vi "Auth Check & Log.vi"(8 "error in":errorcluster, 10 "User Cred":T1, 11 "Authenticated Data":string[][](array[string])) -> (0 "error out":errorcluster, 1 "User":string, 2 "Role Out":string, 3 "Verify Auth":bool)   [LabVIEW 2022 SP3]
uses:
  <vilib>/Utility/file.llb/Write Delimited Spreadsheet (string).vi
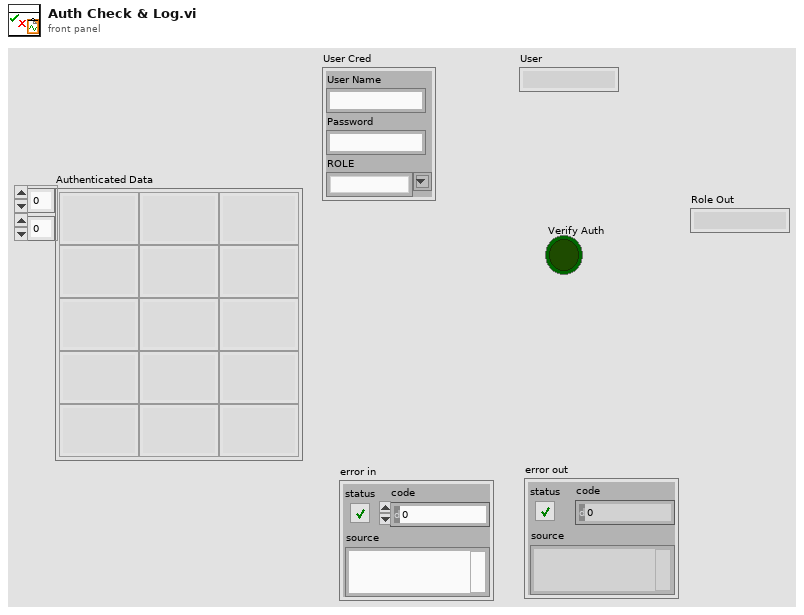
[diagram p1: front panel]
types:
  T1 = cluster{"User Name":string, "Password":string, "ROLE":string}
  T2 = typedef "SeCrTs-file folder ctl.ctl" = cluster{"Datalog path":path, "Configuration path":path, "Signal list path":path, "Sub vi's":path, "Authentication":path, "Sequence":path, "Event Log":path, "CS Error log":path, "RT Error Log":path}
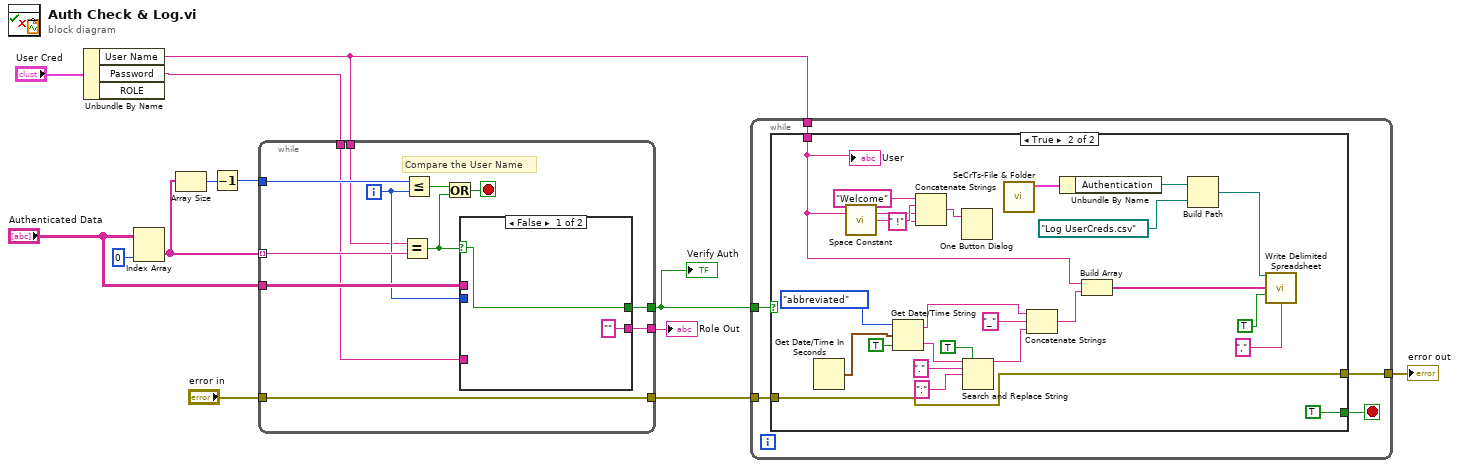
[diagram p0: block diagram]
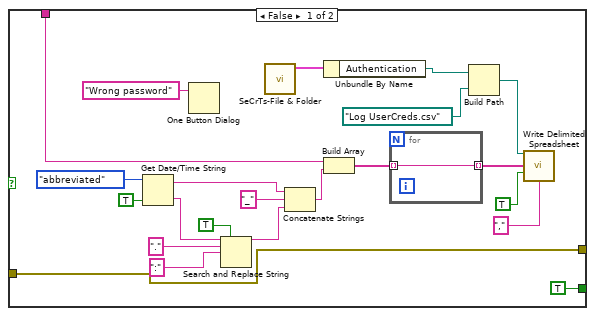
[diagram p2: hidden frame]
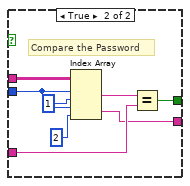
[diagram p3: hidden frame]
diagram:
  n1 = Unbundle By Name("User Cred") -> ("User Name"=w8:string, "Password"=w7:string)  [unwired: 1 out]
  n2 = Index Array(array="Authenticated Data", index (col)=0 ("disabled index (col)")) -> (element=w10:string[])  [unwired: 1 in]
  n3 = Array Size(array=w10) -> (size(s)=w12:i32)
  n4 = Decrement(x=w12) -> (x-1=w11:i32)
  n5 = while {
    tunnel: w11 -> [w25]
    tunnel: w10 -> [w24] mode=indexing
    tunnel: "Authenticated Data" -> [w20]
    tunnel: [w18] -> w9
    tunnel: w8 -> [w16]
    tunnel: w7 -> [w17]
    tunnel: "error in" -> [w15]
    tunnel: [w15] -> w5
    tunnel: [w14] -> w1
    i -> [w19]
    stop <- w21 stop-if-true
    # "Compare the User Name"
    n6 = Equal?(x=w16, y=w24) -> (x = y?=w22:bool)
    n7 = Less Or Equal?(x=w25, y=w19) -> (x <= y?=w23:bool)
    n8 = Or(x=w23, y=w22) -> (x .or. y?=w21:bool)
    n9 = case shown="False" w22 {
      selector: w22 -> [w27 _]
      tunnel: w20 -> [_ w35]
      tunnel: w19 -> [_ w29]
      tunnel: [w27 w32] -> w18
      tunnel: w17 -> [_ w31]
      tunnel: ["" ("String") w28] -> w14
      frame False {
      }
      frame True {
        # "Compare the Password"
        n10 = Index Array(array=w35, index (row) #1=w29, index (col) #1=1 ("disabled index (col)"), index (row) #2=w29, index (col) #2=2 ("index (col)")) -> (element #1=w33:string, element #2=w28:string)
        n11 = Equal?(x=w33, y=w31) -> (x = y?=w32:bool)
      }
    }
  }
  "Verify Auth" <- w9
  "Role Out" <- w1
  n12 = while {
    tunnel: w9 -> [w40]
    tunnel: w8 -> [w38]
    tunnel: w5 -> [w37]
    tunnel: [w36] -> w4
    stop <- w39 stop-if-true
    n13 = case shown="True" w40 {
      tunnel: [TRUE TRUE] -> w39
      tunnel: w38 -> [w44 w65]
      tunnel: w37 -> [w45 w72]
      tunnel: [w45 w72] -> w36
      frame False {
        # "Log user credentials including username,Password and  login time"
        n14 = Get Date/Time String(date format (0)=enum16{"short", "long", "abbreviated"}."abbreviated", want seconds? (F)=TRUE) -> (date string=w60:string, time string=w58:string)  [unwired: 1 in]
        n15 = One Button Dialog(message="Wrong password") -> ()  [unwired: 1 in, 1 out]
        n16 = Search and Replace String(replace all?=TRUE ("replace all? (F)"), input string=w58, search string=".", replace string=":" ("replace string (\"\")")) -> (result string=w59:string)  [unwired: 4 in, 3 out]
        n17 = call "SeCrTs-File & Folder.vi"() -> ("File Output"=w41:T2)  [unwired: 10 in, 1 out]
        n18 = Concatenate Strings(w60, "_" ("string"), w59) -> (w43:string)
        n19 = Unbundle By Name(w41) -> ("Authentication"=w42:path)
        n20 = Build Array(w44, w43) -> (w61:string[])
        n21 = for {
          tunnel: w61 -> [w63] mode=indexing
          tunnel: [w63] -> w62 mode=indexing
        }
        n22 = Build Path(base path=w42, name or relative path=path "Log UserCreds.csv") -> (appended path=w46:path)
        n23 = call-poly <vilib>:"Write Delimited Spreadsheet.vi"("file path (dialog if empty)"=w46, "1D data"=w62, "append to file? (new file:F)"=TRUE, "delimiter (\\t)"="," ("delimiter (\\t)")) -> ()  [unwired: 10 in, 2 out]
      }
      frame True {
        # "Log user credentials including username,Password and  login time"
        n24 = Get Date/Time In Seconds() -> (seconds since 1Jan1904=w64:timestamp)
        n25 = call <vilib>:"Space Constant.vi"() -> ("String"=w68:string)
        n26 = Get Date/Time String(date format (0)=enum16{"short", "long", "abbreviated"}."abbreviated", seconds (now)=w64, want seconds? (F)=TRUE) -> (date string=w81:string, time string=w86:string)
        n27 = Concatenate Strings("Welcome", w68, w65, " !" ("string")) -> (w66:string)
        n28 = One Button Dialog(message=w66) -> ()  [unwired: 1 in, 1 out]
        n29 = Search and Replace String(replace all?=TRUE ("replace all? (F)"), input string=w86, search string=".", replace string=":" ("replace string (\"\")")) -> (result string=w83:string)  [unwired: 4 in, 3 out]
        n30 = call "SeCrTs-File & Folder.vi"() -> ("File Output"=w70:T2)  [unwired: 10 in, 1 out]
        n31 = Concatenate Strings(w81, "_" ("string"), w83) -> (w79:string)
        n32 = Unbundle By Name(w70) -> ("Authentication"=w71:path)
        n33 = Build Array(w65, w79) -> (w78:string[])
        n34 = Build Path(base path=w71, name or relative path=path "Log UserCreds.csv") -> (appended path=w73:path)
        n35 = call-poly <vilib>:"Write Delimited Spreadsheet.vi"("file path (dialog if empty)"=w73, "1D data"=w78, "append to file? (new file:F)"=TRUE, "delimiter (\\t)"="," ("delimiter (\\t)")) -> ()  [unwired: 10 in, 2 out]
        "User" <- w65
      }
    }
  }
  "error out" <- w4
